vi "led wave.vi"() -> ()   [LabVIEW 2019]
uses:
  <vilib>/Rock Robotics/SystemInterfaces/DIO/FPGA_DIOPWMChannel.ctl
panel:
  in  "Color Box 2":u32(colorbox)=15663126
  in  "Color Box":u32(colorbox)=15663126
  in  "PWM Channel":T1=enum."PWM 9"
  in  "String Length":u32=8
  in  "stop":bool
  out "LED Strip":u32[](array[colorbox])
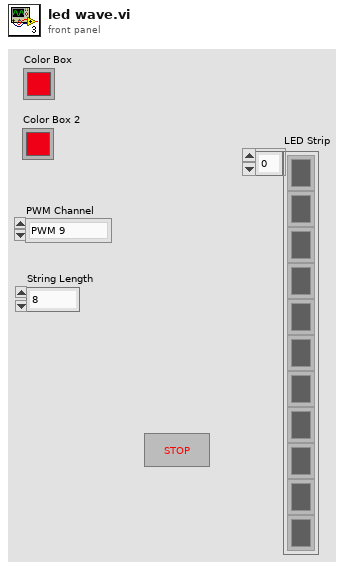
[diagram p1: front panel]
types:
  T1 = typedef "FPGA_DIOPWMChannel.ctl" = enum8{"PWM 0", "PWM 1", "PWM 2", "PWM 3", "PWM 4", "PWM 5", "PWM 6", "PWM 7", "PWM 8", "PWM 9", "PWM MXP 0", "PWM MXP 1", "PWM MXP 2", "PWM MXP 3", "PWM MXP 4", "PWM MXP 5", "PWM MXP 6", "PWM MXP 7", "PWM MXP 8", "PWM MXP 9", "Invalid"}
  T2 = typedef "WPI_PWMDeviceRef.ctl" = cluster{"DeviceStatus":errorcluster, "PWM Channel":T1}
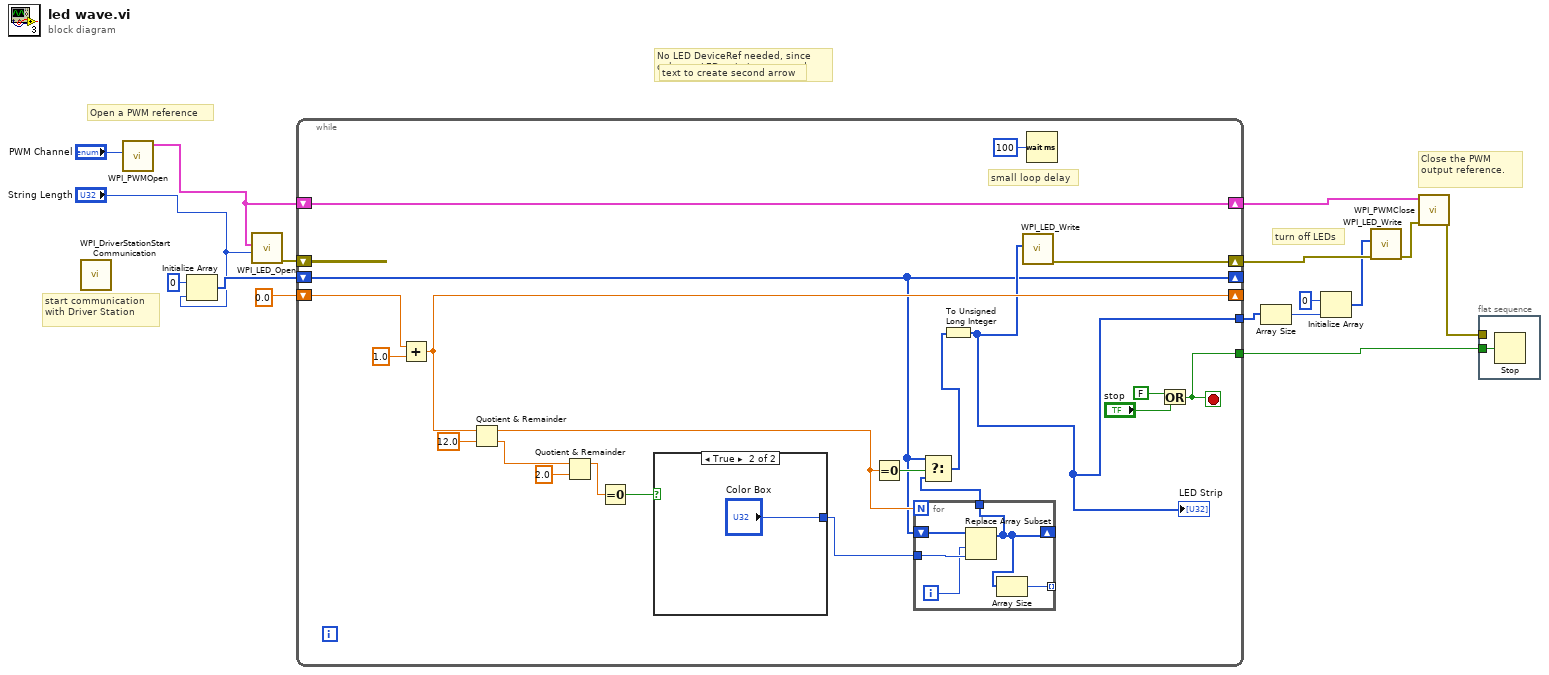
[diagram p0: block diagram]
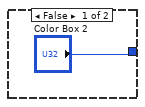
[diagram p2: hidden frame]
diagram:
  # "Open a PWM reference"
  # "start communication with Driver Station"
  # "turn off LEDs"
  # "No LED DeviceRef needed, since only one LED strip is supported"
  # "Close the PWM output reference."
  # "text to create second arrow"
  n1 = call <vilib>:"WPI_DriverStationStart Communication.vi"() -> ()  [unwired: 2 in, 10 out]
  n2 = call <vilib>:"WPI_PWMOpen.vi"("PWM Channel"="PWM Channel") -> ("PWMDeviceRef"=w5:T2)  [unwired: 9 in, 1 out]
  n3 = Initialize Array(u32 0 ("element"), "String Length") -> (w3:u32[])
  n4 = call <vilib>:"WPI_LED_Open.vi"("String Length"="String Length", "PWMDeviceRef"=w5) -> ("error out"=w14:errorcluster)  [unwired: 9 in]
  n5 = while {
    shift-right: [w34] -> w15
    shift-left: w5 -> [w34]
    tunnel: [w36] -> w16
    shift-right: [w33] -> w13
    shift-left: w14 -> [_]
    tunnel: [w22] -> w10
    shift-right: [w30] -> _
    shift-left: 0.0 -> [w31]
    shift-right: [w19] -> _
    shift-left: w3 -> [w19]
    stop <- w36 stop-if-true
    # "small loop delay"
    n6 = Add(x=w31, y=1.0) -> (x+y=w30:dbl)
    n7 = Quotient & Remainder(x=w30, y=12.0) -> (x-y*floor(x/y)=w20:dbl, floor(x/y)=w27:dbl)
    n8 = Quotient & Remainder(x=w27, y=2.0) -> (x-y*floor(x/y)=w24:dbl)  [unwired: 1 out]
    n9 = Equal To 0?(x=w24) -> (x = 0?=w25:bool)
    n10 = case shown="True" w25 {
      tunnel: ["Color Box 2" "Color Box"] -> w23
      frame False {
      }
      frame True {
      }
    }
    n11 = Equal To 0?(x=w20) -> (x = 0?=w21:bool)
    n12 = for {
      N: w20 -> [_]
      tunnel: w23 -> [w42]
      tunnel: [w39] -> w18
      shift-right: [w39] -> _
      shift-left: w19 -> [w41]
      tunnel: [w38] -> _ mode=indexing
      i -> [w40]
      n13 = Replace Array Subset(array=w41, new element=w42, index=w40) -> (w39:u32[])
      n14 = Array Size(array=w39) -> (size(s)=w38:i32)
    }
    n15 = Select(t=w19, s=w21, f=w18) -> (s? t:f=w17:u32[])
    n16 = To Unsigned Long Integer(number=w17) -> (unsigned 32bit integer=w22:u32[])
    "LED Strip" <- w22
    n17 = call <vilib>:"WPI_LED_Write.vi"("Color Array"=w22) -> ("error out"=w33:errorcluster)  [unwired: 10 in]
    n18 = Wait (ms)(milliseconds to wait=u32 100) -> ()  [unwired: 1 out]
    n19 = Or(x=FALSE, y="stop") -> (x .or. y?=w36:bool)
  }
  n20 = Array Size(array=w10) -> (size(s)=w11:i32)
  n21 = Initialize Array(u32 0, w11) -> (w8:u32[])
  n22 = call <vilib>:"WPI_LED_Write.vi"("error in"=w13, "Color Array"=w8) -> ("error out"=w12:errorcluster)  [unwired: 9 in]
  n23 = call <vilib>:"WPI_PWMClose.vi"("error in (no error)"=w12, "PWMDeviceRef"=w15) -> ("error out"=w7:errorcluster)  [unwired: 9 in]
  n24 = flat-sequence {
    tunnel: w16 -> [w45]
    tunnel: w7 -> [_]
    frame #0 {
      n25 = Stop(stop? (T)=w45) -> ()
    }
  }
